vi "Construct.vi"(8 "error in (no error)":errorcluster, 11 "CDependencyList in":refnum<class "CDependencyList.lvclass">) -> (0 "error out":errorcluster, 3 "CDependencyList out":refnum<class "CDependencyList.lvclass">)   [LabVIEW 2020, in "DependencyInspection.lvlib" / "CDependencyList.lvclass"]
uses:
  CDependencyList.lvclass
  DependencyList.ctl
  obj/Addons/LabVIEWObjectInterfaces.lvlibp/LabVIEWObjectInterfaces/ILabVIEWItem/ILabVIEWItem.lvclass
  QualifiedNamesToPathsMap.ctl
  CDependencyList.lvclass/CDependencyList.ctl
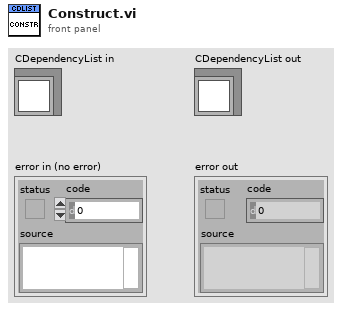
[diagram p1: front panel]
types:
  T1 = typedef "DependencyInspection.lvlib/CDependencyList.lvclass/QualifiedNamesToPathsMap.ctl" = map{string, string}
  T2 = typedef "DependencyInspection.lvlib/CDependencyList.lvclass/DependencyList.ctl" = map{string, refnum<class "ILabVIEWItem.lvclass">}
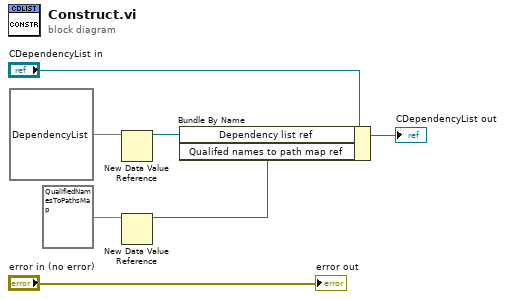
[diagram p0: block diagram]
diagram:
  n1 = New Data Value Reference(data value=T2 {} ("Dependency List")) -> (data value reference=w4:refnum<data-value>)  [unwired: 1 in, 1 out]
  n2 = New Data Value Reference(data value=T1 {} ("Qualified names to paths")) -> (data value reference=w1:refnum<data-value>)  [unwired: 1 in, 1 out]
  n3 = Bundle By Name(cluster="CDependencyList in", "Dependency list ref"=w4, "Qualifed names to path map ref"=w1) -> (→"CDependencyList out":refnum<class "CDependencyList.lvclass">)
  "error out" <- "error in (no error)"
